vi "Generate Pinmap.vi"(10 "grpc-labview code gen path":path=path "C:/Program Files/National Instruments/LabVIEW 2020/vi.lib/gRPC/gRPC Server and Client Template [2]/gRPC Scripting Tools/Main.vi", 11 "pinmap generation params":T1={"Proto File Path"=[path "Protos/ni/measurementlink/pinmap/v1/pin_map_service.proto"], "Import Paths"=[path "Protos"], "Prototype Library"=path "Runtime/Pin Map Client Prototype Library.lvlib", "Target Project"=path "Runtime/Pin Map Client.lvproj", "Target Name"="My Computer", "Generated Library Name"="MeasurementLink Pin Map", "Library Suffix"=" Client", "Generate"=enum."gRPC Client"}) -> (0 "error out":errorcluster)   [LabVIEW 2020]
uses:
  grpc-labview Template Options.ctl
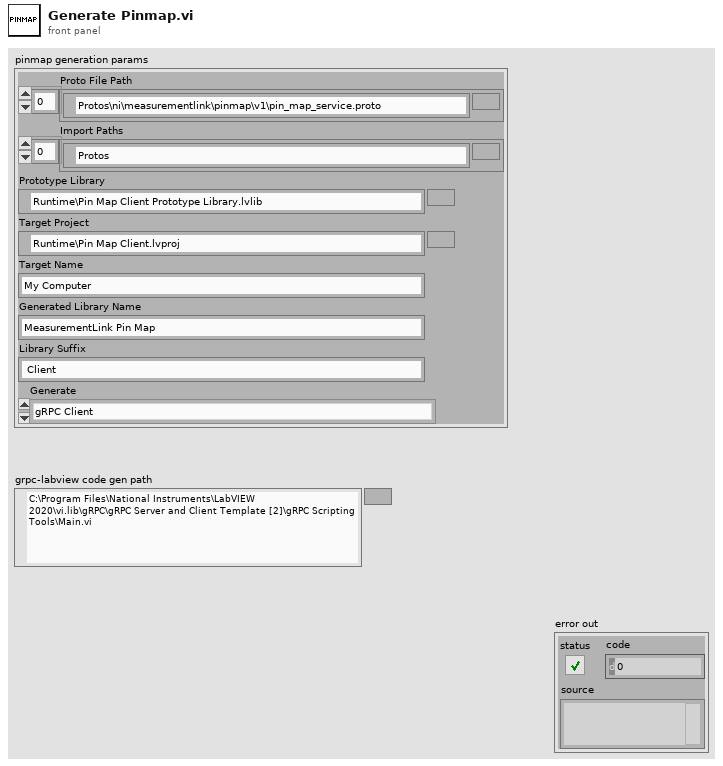
[diagram p1: front panel]
types:
  T1 = typedef "grpc-labview Template Options.ctl" = cluster{"Proto File Path":path[], "Import Paths":path[], "Prototype Library":path, "Target Project":path, "Target Name":string, "Generated Library Name":string, "Library Suffix":string, "Generate":enum16{"gRPC Server", "gRPC Client", "Both"}}
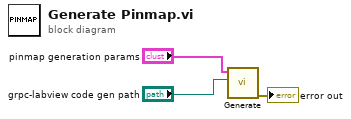
[diagram p0: block diagram]
diagram:
  n1 = call "Generate.vi"("grpc-labview code gen path"="grpc-labview code gen path", "grpc-labview generation params"="pinmap generation params") -> ("error out"=→"error out":errorcluster)  [unwired: 9 in]
